vi "Initialise.vi"(6 "Diffuse Colour":refnum<vi>, 8 "error in (no error)":errorcluster, 9 "Objects":T1[](array[typedef]) {"Triangles"."Vertex 3"."UV"."v" min=0 max=1 step=0.1; "Triangles"."Vertex 3"."UV"."u" min=0 max=1 step=0.1; "Triangles"."Vertex 2"."UV"."v" min=0 max=1 step=0.1; "Triangles"."Vertex 2"."UV"."u" min=0 max=1 step=0.1; "Triangles"."Vertex 1"."UV"."v" min=0 max=1 step=0.1; "Triangles"."Vertex 1"."UV"."u" min=0 max=1 step=0.1}, 11 "Screen Dimensions":T8={"Width"=800, "Height"=600}) -> (0 "error out":errorcluster, 3 "Scene out":refnum<class "Scene.lvclass">)   [LabVIEW 2020, in "Scene.lvclass"]
uses:
  Scene.lvclass
  Scene.lvclass/Scene.ctl
  Graphics/Libraries/3D/3D.lvlib
  Graphics/Libraries/3D/Camera.ctl
  Camera.ctl
  Graphics/Libraries/Raster/Rectangle Dimensions.ctl
  Graphics/Libraries/Raster/Raster.lvlib
  Graphics/Libraries/3D/Vector 3D.ctl
  Graphics/Libraries/Raster/UV.ctl
  Graphics/Libraries/3D/Vertex.ctl
  Graphics/Libraries/Raster/Texture.ctl
  Graphics/Libraries/3D/Material.ctl
  Graphics/Libraries/3D/Triangle.ctl
  Graphics/Libraries/3D/Transform.ctl
  Graphics/Libraries/3D/Object.ctl
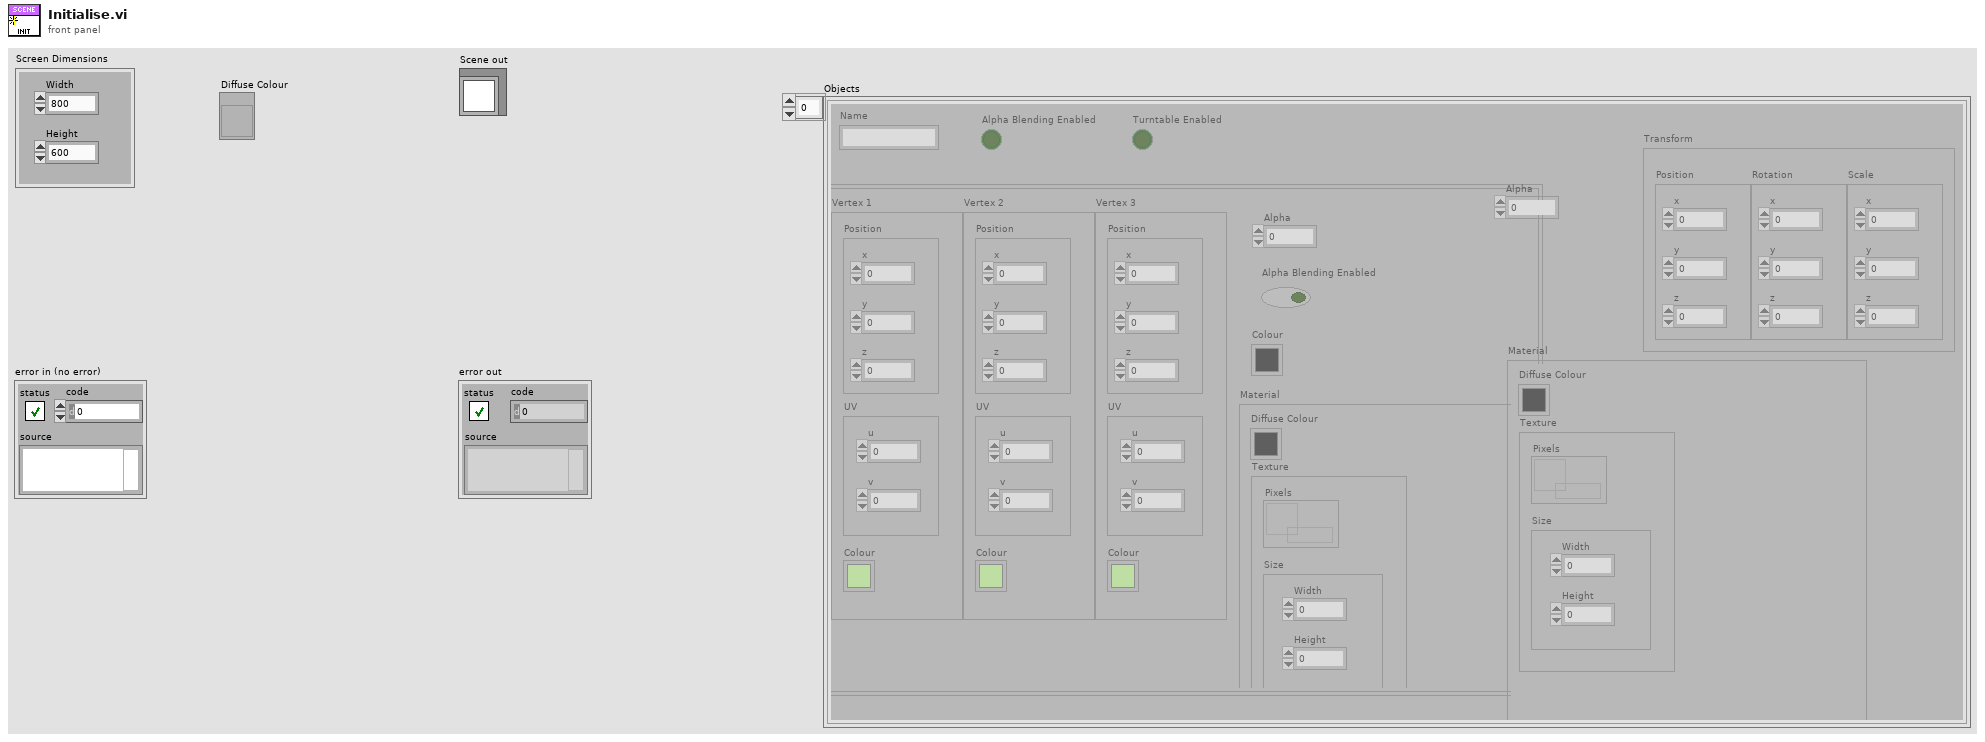
[diagram p1: front panel]
types:
  T1 = typedef "3D.lvlib/Object.ctl" = cluster{"Triangles":T2[], "Transform":T9, "Name":string, "Alpha Blending Enabled":bool, "Alpha":dbl, "Turntable Enabled":bool, "Material":T6}
  T2 = typedef "3D.lvlib/Triangle.ctl" = cluster{"Vertex 1":T3, "Vertex 2":T3, "Vertex 3":T3, "Alpha":dbl, "Alpha Blending Enabled":bool, "Colour":u32, "Material":T6}
  T3 = typedef "3D.lvlib/Vertex.ctl" = cluster{"Position":T4, "UV":T5, "Colour":u32}
  T4 = typedef "3D.lvlib/Vector 3D.ctl" = cluster{"x":sgl, "y":sgl, "z":sgl}
  T5 = typedef "Raster.lvlib/UV.ctl" = cluster{"u":sgl, "v":sgl}
  T6 = typedef "3D.lvlib/Material.ctl" = cluster{"Diffuse Colour":u32, "Texture":T7}
  T7 = typedef "Raster.lvlib/Texture.ctl" = cluster{"Pixels":refnum<data-value>, "Size":T8}
  T8 = typedef "Raster.lvlib/Rectangle Dimensions.ctl" = cluster{"Width":u32, "Height":u32}
  T9 = typedef "3D.lvlib/Transform.ctl" = cluster{"Position":T4, "Rotation":T4, "Scale":T4}
  T10 = typedef "Scene.lvclass/Camera.ctl" = cluster{"Up":sgl, "Left":sgl, "Rotation":sgl, "Forward":sgl}
  T11 = typedef "3D.lvlib/Camera.ctl" = cluster{"Field Of View":sgl, "Near Plane":sgl, "Far Plane":sgl}
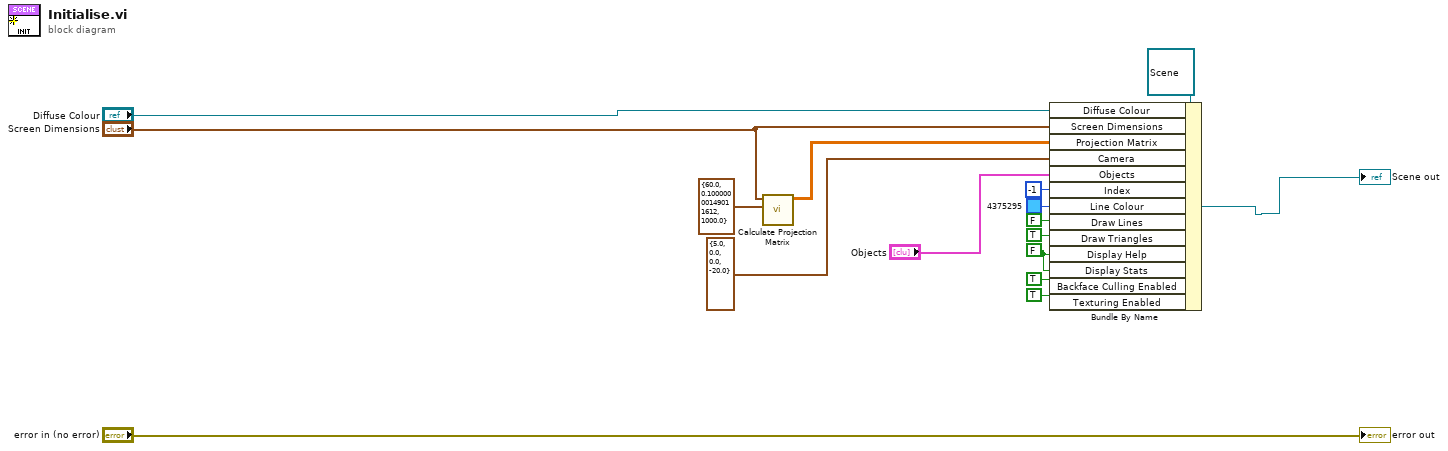
[diagram p0: block diagram]
diagram:
  w6 = FALSE ("Display Help")
  n1 = call "Calculate Projection Matrix.vi"("Camera"=T11 {"Field Of View"=60.0, "Near Plane"=0.1, "Far Plane"=1000.0}, "Screen Dimensions"="Screen Dimensions") -> ("Projection Matrix"=w13:sgl[][])  [unwired: 9 in]
  n2 = Bundle By Name(cluster=refnum<class "Scene.lvclass"> refnum ("Scene in"), "Diffuse Colour"="Diffuse Colour", "Screen Dimensions"="Screen Dimensions", "Projection Matrix"=w13, "Camera"=T10 {"Up"=5.0, "Left"=0.0, "Rotation"=0.0, "Forward"=-20.0}, "Objects"="Objects", "Index"=-1 ("Active Object"), "Line Colour"=u32 4375295, "Draw Lines"=FALSE, "Draw Triangles"=TRUE, "Display Help"=w6, "Display Stats"=w6, "Backface Culling Enabled"=TRUE ("Display Help"), "Texturing Enabled"=TRUE) -> (→"Scene out":refnum<class "Scene.lvclass">)
  "error out" <- "error in (no error)"
